vi "sp_String to 1D String.vi"(0 "script":string, 1 "seperator":string="\n", 11 "error in (no error)":errorcluster) -> (4 "Script Lines":string[](array[string]), 15 "error out":errorcluster)   [LabVIEW 2019]
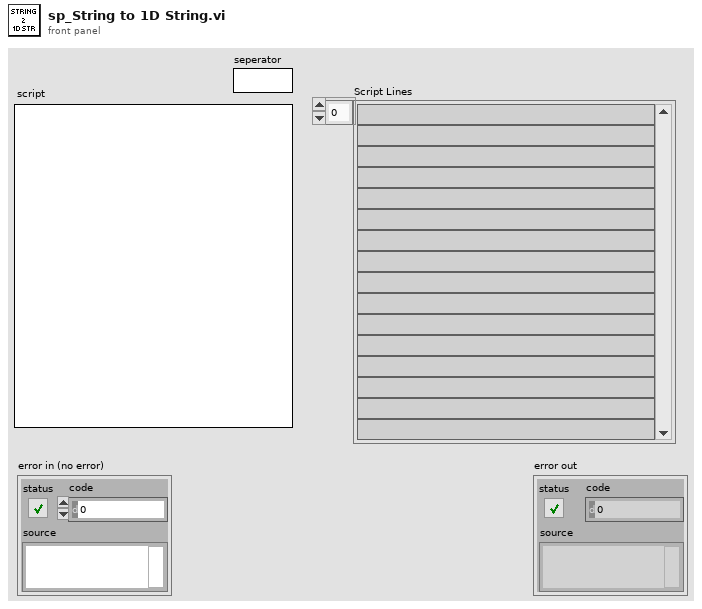
[diagram p1: front panel]
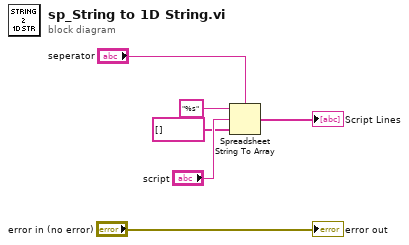
[diagram p0: block diagram]
diagram:
  n1 = Spreadsheet String To Array(delimiter (Tab)="seperator", format string="%s", spreadsheet string="script", array type (2D Dbl)=string[] []) -> (array=→"Script Lines":string[])
  "error out" <- "error in (no error)"
